vi "SSL_CTX_new.vi"(8 "error in (no error)":errorcluster, 10 "*SSL_Method":u64, 11 "SSL-Lib in":refnum<class "SSL-Lib.lvclass">) -> (0 "error out":errorcluster, 2 "SSL-Context out":refnum<class "SSL-Context.lvclass">, 3 "SSL-Lib out":refnum<class "SSL-Lib.lvclass">)   [LabVIEW 2013, in "SSL_Lib.lvlib" / "SSL-Lib.lvclass"]
uses:
  SSL-Lib.lvclass
  SSL-Context/SSL-Context.lvclass
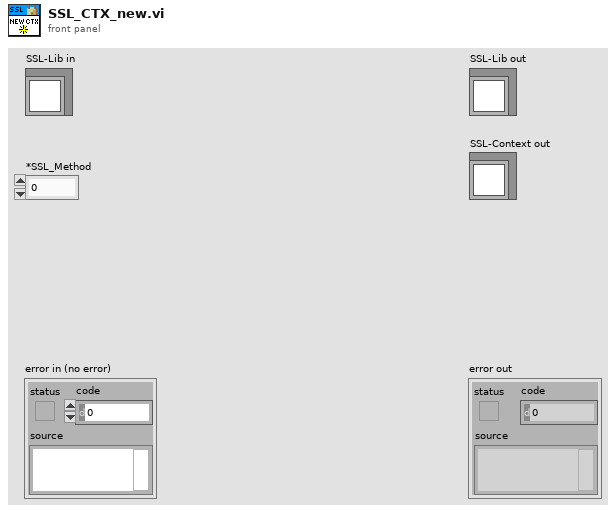
[diagram p1: front panel]
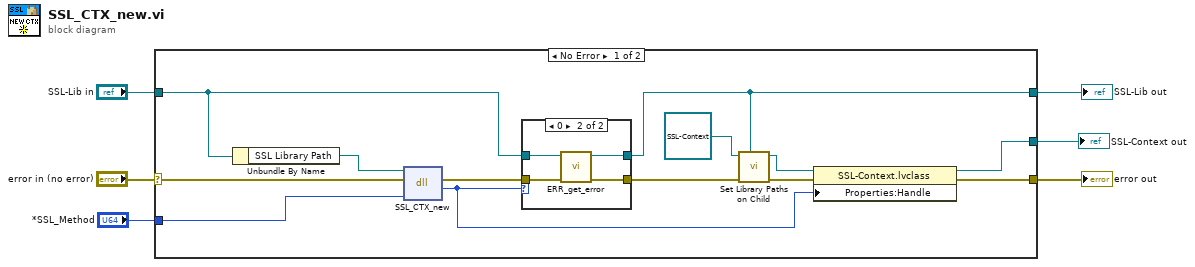
[diagram p0: block diagram]
diagram:
  n1 = case shown="No Error" "error in (no error)" {
    selector: "error in (no error)" -> [w19 w27]
    tunnel: [w12 w27] -> w5
    tunnel: [w9 w26] -> w3
    tunnel: "SSL-Lib in" -> [w10 w26]
    tunnel: "*SSL_Method" -> [w17 _]
    tunnel: [w16 _] -> w1
    frame No Error {
      n2 = Unbundle By Name(w10) -> ("SSL Library Path"=w18:path)
      n3 = dll-call lib="C:/Program Files (x86)/National Instruments/Shared/nissl/NIssleay32.dll" fn="SSL_CTX_new"(path in=w18, error in=w19, "SSL_Method"=w17) -> (error out=w11:errorcluster, "return type"=w7:u64)  [unwired: 2 in, 1 out]
      n4 = case shown="0" w7 {
        tunnel: w11 -> [w21 w25]
        tunnel: w10 -> [w20 w24]
        tunnel: [w20 w23] -> w9
        tunnel: [w21 w22] -> w8
        frame Default {
        }
        frame 0 {
          n5 = call "ERR_get_error.vi"("error in (no error)"=w25, "SSL-Lib in"=w24) -> ("error out"=w22:errorcluster, "SSL-Lib out"=w23:refnum<class "SSL-Lib.lvclass">)  [unwired: 8 in]
        }
      }
      n6 = call-dynamic "Set Library Paths on Child.vi"(7:"SSL-Lib in"=w9, "error in (no error)"=w8, 11:"SSL-Lib in"=refnum<class "SSL-Context.lvclass"> refnum ("SSL-Lib.lvlib:SSL-Context.lvclass")) -> ("error out"=w13:errorcluster, "SSL-Lib out"=w14:refnum<class "SSL-Context.lvclass">)  [unwired: 7 in]
      n7 = property class="SSL-Context.lvclass"(reference=w14, error in=w13, "Properties:Handle"=w7) -> (reference out=w16:refnum<class "SSL-Context.lvclass">, error out=w12:errorcluster)
    }
    frame Error {
    }
  }
  "error out" <- w5
  "SSL-Lib out" <- w3
  "SSL-Context out" <- w1
